vi "Write Field (String).vi"(7 "field name":string, 8 "error in":errorcluster, 10 "value":string, 11 "PV Data in":refnum<class "PV Data.lvclass">) -> (0 "error out":errorcluster, 2 "value out":string, 3 "PV Data out":refnum<class "PV Data.lvclass">)   [LabVIEW 2020, in "PV Access.lvlib" / "PV Data.lvlib" / "PV Data.lvclass"]
uses:
  PV Data.lvclass
  PV Access.lvlib
  <vilib>/addons/Tools/Unicode/UTF8 Tools.lvlib
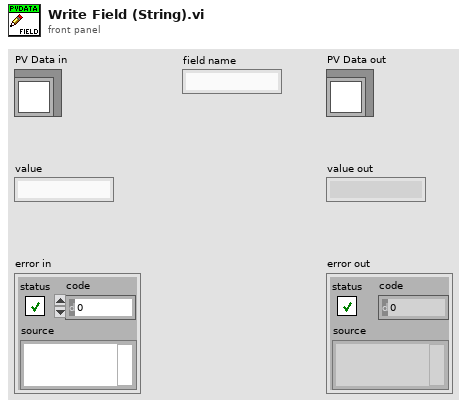
[diagram p1: front panel]
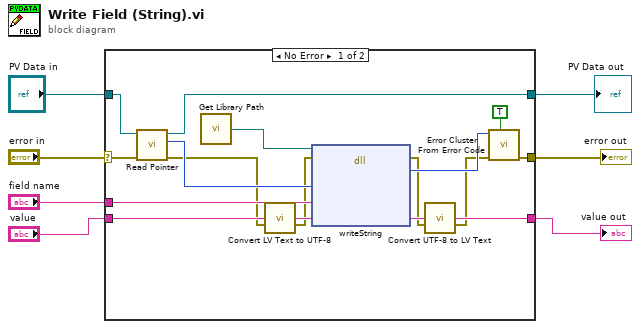
[diagram p0: block diagram]
diagram:
  n1 = case shown="No Error" "error in" {
    selector: "error in" -> [w17 w27]
    tunnel: [w19 w27] -> w7
    tunnel: "value" -> [w24 w26]
    tunnel: [w23 w26] -> w4
    tunnel: [w16 w25] -> w2
    tunnel: "PV Data in" -> [w18 w25]
    tunnel: "field name" -> [w14 _]
    frame No Error {
      n2 = call-dynamic "Read Pointer.vi"("error in (no error)"=w17, "Pointer Base in"=w18) -> ("error out"=w11:errorcluster, "Pointer"=w15:i64, "Pointer Base out"=w16:refnum<class "PV Data.lvclass">)  [unwired: 7 in]
      n3 = call "Get Library Path.vi"() -> ("Path"=w22:path)  [unwired: 1 in]
      n4 = call <vilib>:"Convert LV Text to UTF-8.vi"("LV Text"=w24, "error in"=w11) -> ("UTF-8 Text"=w13:string, "error out"=w10:errorcluster)  [unwired: 12 in]
      n5 = dll-call lib="?" fn="writeString"(path in=w22, error in=w10, "value"=w15, "field_name"=w14, "new_value"=w13) -> (error out=w9:errorcluster, "err_code"=w20:i32, "new_value"=w12:string)  [unwired: 3 in, 1 out]
      n6 = call <vilib>:"Convert UTF-8 to LV Text.vi"("UTF-8 Text"=w12, "error in"=w9) -> ("LV Text"=w23:string, "error out"=w8:errorcluster)  [unwired: 12 in]
      n7 = call <vilib>:"Error Cluster From Error Code.vi"("show call chain? (False)"=TRUE, "error in (no error)"=w8, "error code (0)"=w20) -> ("error out"=w19:errorcluster)  [unwired: 6 in]
    }
    frame Error {
    }
  }
  "error out" <- w7
  "value out" <- w4
  "PV Data out" <- w2
